vi "Configure - DML.vi"(8 "error in (no error)":errorcluster, 11 "DriveMotors in":refnum<class "DriveMotors.lvclass">) -> (0 "error out":errorcluster, 3 "DriveMotors out":refnum<class "DriveMotors.lvclass">)   [LabVIEW 2013]
uses:
  Systems/DriveMotors/DriveMotors.lvclass
  <vilib>/Utility/config.llb/Read Key (Double).vi
  <vilib>/Utility/config.llb/Write Key (Double).vi
  <vilib>/Utility/config.llb/NI_LVConfig.lvlib
panel:
  in  "Encoder Maximum Rate":dbl=5000.0
  in  "Wheel diameter (in)":dbl=6.0
  in  "Encoder DistancePerCount (deg)":dbl=1.40625
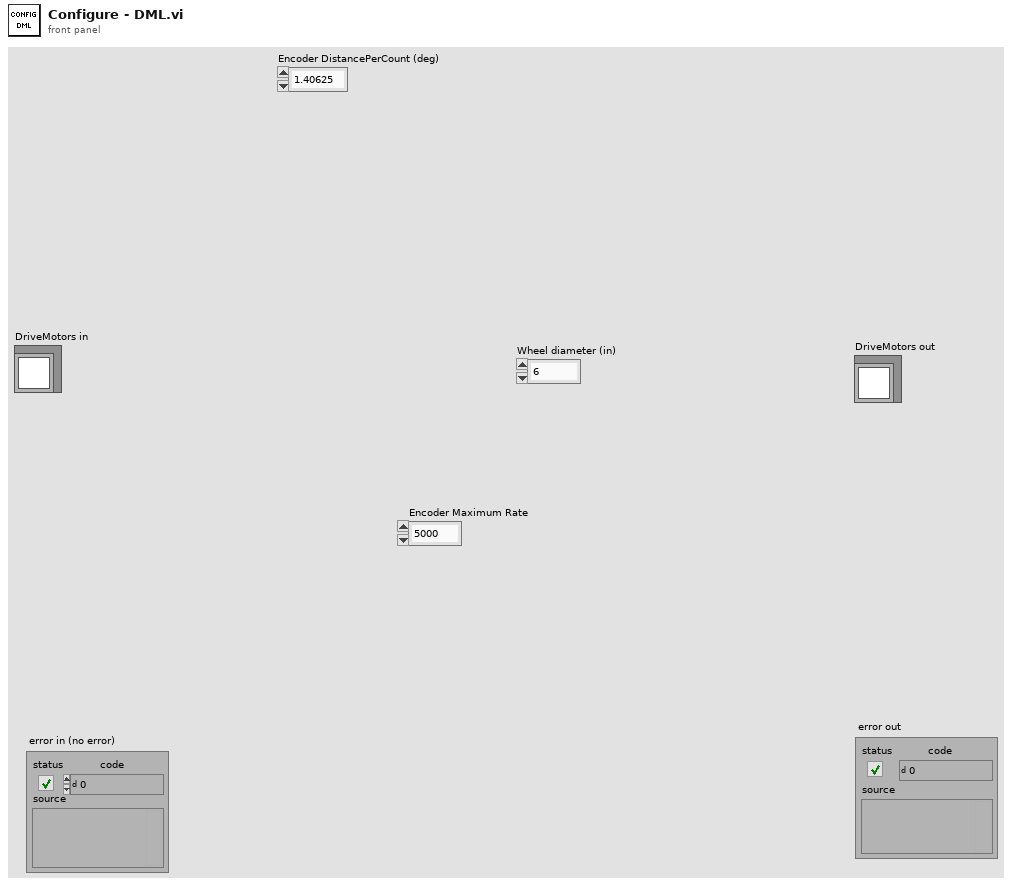
[diagram p1: front panel]
types:
  T1 = typedef "NI_LVConfig.lvlib/Config Data RefNum.ctl" = refnum<k1>
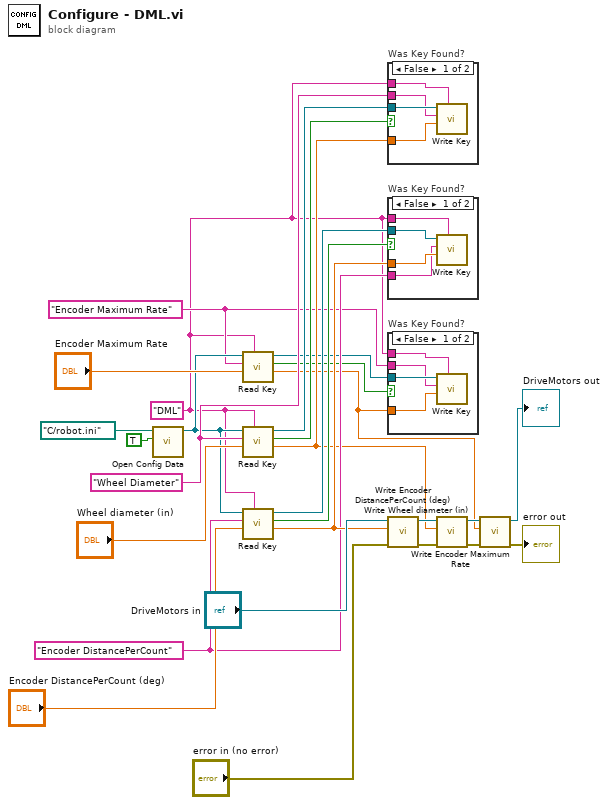
[diagram p0: block diagram]
diagram:
  w4 = "Encoder Maximum Rate" ("key")
  w9 = "Wheel Diameter" ("key")
  w3 = "DML" ("section")
  w13 = "Encoder DistancePerCount" ("key")
  n1 = call <vilib>:"Open Config Data.vi"("create file if necessary (T)"=TRUE, "configuration file path"=path "C:/robot.ini") -> ("refnum"=w6:T1)  [unwired: 7 in, 2 out]
  n2 = call-poly <vilib>:"Read Key.vi"("section"=w3, "default value"="Encoder Maximum Rate", "key"=w4, "refnum"=w6) -> ("value"=w2:dbl, "found?"=w1:bool, "refnum out"=w5:T1)  [unwired: 4 in, 1 out]
  n3 = call-poly <vilib>:"Read Key.vi"("section"=w3, "default value"="Wheel diameter (in)", "key"=w9, "refnum"=w6) -> ("value"=w8:dbl, "found?"=w11:bool, "refnum out"=w10:T1)  [unwired: 4 in, 1 out]
  n4 = call-poly <vilib>:"Read Key.vi"("section"=w3, "default value"="Encoder DistancePerCount (deg)", "key"=w13, "refnum"=w6) -> ("value"=w15:dbl, "found?"=w16:bool, "refnum out"=w14:T1)  [unwired: 4 in, 1 out]
  n5 = case "Was Key Found?" shown="False" w11 {
    tunnel: w10 -> [w31 _]
    tunnel: w9 -> [w30 _]
    tunnel: w8 -> [w29 _]
    tunnel: w3 -> [w28 _]
    frame False {
      n6 = call-poly <vilib>:"Write Key.vi"("section"=w28, "value"=w29, "key"=w30, "refnum"=w31) -> ()  [unwired: 5 in, 3 out]
    }
    frame True {
    }
  }
  n7 = case "Was Key Found?" shown="False" w16 {
    tunnel: w15 -> [w35 _]
    tunnel: w3 -> [w34 _]
    tunnel: w14 -> [w33 _]
    tunnel: w13 -> [w32 _]
    frame False {
      n8 = call-poly <vilib>:"Write Key.vi"("section"=w34, "value"=w35, "key"=w32, "refnum"=w33) -> ()  [unwired: 5 in, 3 out]
    }
    frame True {
    }
  }
  n9 = case "Was Key Found?" shown="False" w1 {
    tunnel: w5 -> [w39 _]
    tunnel: w4 -> [w38 _]
    tunnel: w3 -> [w37 _]
    tunnel: w2 -> [w36 _]
    frame False {
      n10 = call-poly <vilib>:"Write Key.vi"("section"=w37, "value"=w36, "key"=w38, "refnum"=w39) -> ()  [unwired: 5 in, 3 out]
    }
    frame True {
    }
  }
  n11 = call-dynamic "Write Encoder DistancePerCount (deg).vi"("error in (no error)"="error in (no error)", "Encoder DistancePerCount (deg)"=w15, "DriveMotors in"="DriveMotors in") -> ("error out"=w22:errorcluster, "DriveMotors out"=w24:refnum<class "DriveMotors.lvclass">)  [unwired: 7 in]
  n12 = call-dynamic "Write Wheel diameter (in).vi"("error in (no error)"=w22, "Wheel diameter (in)"=w8, "DriveMotors in"=w24) -> ("error out"=w26:errorcluster, "DriveMotors out"=w27:refnum<class "DriveMotors.lvclass">)  [unwired: 7 in]
  n13 = call-dynamic "Write Encoder Maximum Rate.vi"("error in (no error)"=w26, "Encoder Maximum Rate"=w2, "DriveMotors in"=w27) -> ("error out"=→"error out":errorcluster, "DriveMotors out"=→"DriveMotors out":refnum<class "DriveMotors.lvclass">)  [unwired: 7 in]
